vi "ComboBox - Drop Down Menu.vi"(10 "CtlRef":refnum<vi>, 11 "VI in (This VI)":refnum<vi>) -> (1 "y":u32, 2 "x":u32, 3 "Front Panel Window:Panel Bounds":T2)   [LabVIEW 2013]
uses:
  <vilib>/Utility/miscctls.llb/LVRectTypeDef.ctl
  Controls/Combo Box.ctl
  <vilib>/Utility/miscctls.llb/LVPointTypeDef.ctl
panel:
  in  "ComboBox":T1
  # "These Coordinates will work for this type (size) of ComboBox"
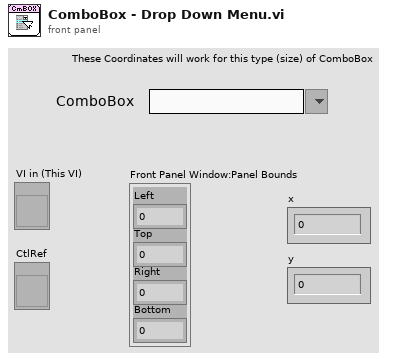
[diagram p1: front panel]
types:
  T1 = typedef "Combo Box.ctl" = string
  T2 = typedef "LVRectTypeDef.ctl" = cluster{"Left":i16, "Top":i16, "Right":i16, "Bottom":i16}
  T3 = typedef "LVPointTypeDef.ctl" = cluster{"Horizontal":i16, "Vertical":i16}
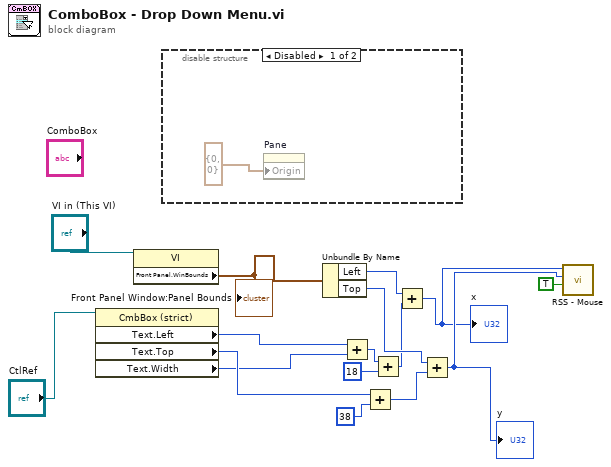
[diagram p0: block diagram]
diagram:
  n1 = property on="Property Node" class="CmbBox (strict)"(reference="CtlRef") -> ("Text.Left"=w1:i32, "Text.Top"=w4:i32, "Text.Width"=w2:u32)  [unwired: 1 in, 2 out]
  n2 = property class="VI"(reference="VI in (This VI)") -> ("Front Panel.WinBounds"=w7:T2)  [unwired: 1 in, 2 out]
  "Front Panel Window:Panel Bounds" <- w7
  n3 = disable-structure shown="Disabled" {
    frame Disabled {
      n4 = property on="Pane" class="Pane"("Origin"=T3 {"Horizontal"=0, "Vertical"=0}) -> ()  [unwired: 2 in, 2 out]
    }
    frame Enabled {
    }
  }
  n5 = Unbundle By Name(w7) -> ("Left"=w8:i16, "Top"=w10:i16)
  n6 = Add(x=w1, y=w2) -> (x+y=w3:u32)
  n7 = Add(x=w4, y=u32 38) -> (x+y=w11:u32)
  n8 = Add(x=w3, y=u32 18) -> (x+y=w9:u32)
  n9 = Add(x=w8, y=w9) -> (x+y=w13:u32)
  "x" <- w13
  n10 = Add(x=w10, y=w11) -> (x+y=w14:u32)
  "y" <- w14
  n11 = call "RSS - Mouse.vi"("Click"=TRUE, "y"=w14, "x"=w13) -> ()  [unwired: 9 in]
